vi "Read Msg Output.vi"(10 "Msg Output":refnum<class "Msg Output.lvclass">) -> (0 "Error out":errorcluster)   [LabVIEW 2025, in "_Template.lvlib" / "Templates.lvlib" / "TEMPLATE Msg.lvlib" / "TEMPLATE Msg Output.lvlib"]
uses:
  TEMPLATE Msg Output.lvlib
  jettl/jettl/Msg Output/Msg Output.lvclass
  TEMPLATE Msg Output/TEMPLATE Msg Output.lvclass
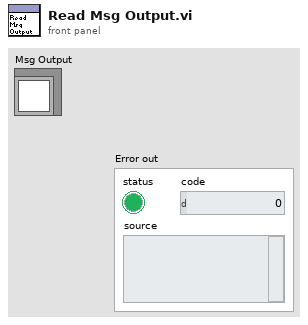
[diagram p1: front panel]
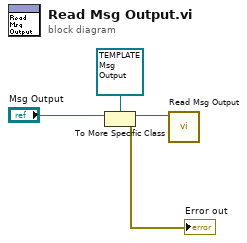
[diagram p0: block diagram]
diagram:
  n1 = To More Specific Class(target class=refnum<class "TEMPLATE Msg Output.lvclass"> refnum ("_Template.lvlib:Templates.lvlib:TEMPLATE Msg.lvlib:TEMPLATE Msg Output.lvclass"), reference="Msg Output") -> (specific class reference=w1:refnum<class "TEMPLATE Msg Output.lvclass">, error out=→"Error out":errorcluster)  [unwired: 1 in]
  n2 = call "Read Msg Output.vi"("TEMPLATE Msg Output in"=w1) -> ()  [unwired: 11 in]
